vi "QinABCDQout.vi"(1 "ABCD":cluster{"A":dbl, "B":dbl, "C":dbl, "D":dbl} {"D" format="%.2f"; "C" format="%.2f"; "B" format="%.2f"; "A" format="%.2f"}, 2 "Q in":cdb format="%.2f") -> (0 "Q out":cdb format="%.2f")   [LabVIEW 2017]
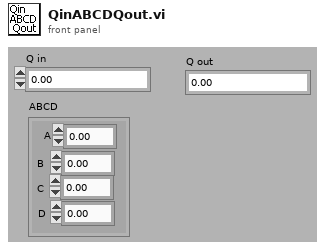
[diagram p1: front panel]
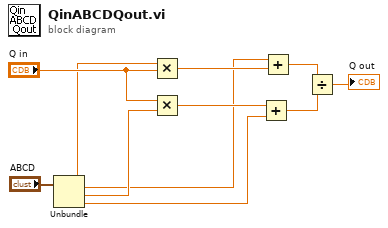
[diagram p0: block diagram]
diagram:
  n1 = Unbundle("ABCD") -> ("A"=w4:dbl, "B"=w2:dbl, "C"=w3:dbl, "D"=w1:dbl)
  n2 = Multiply(x=w4, y="Q in") -> (x*y=w10:cdb)
  n3 = Multiply(x="Q in", y=w3) -> (x*y=w9:cdb)
  n4 = Add(x=w9, y=w1) -> (x+y=w7:cdb)
  n5 = Add(x=w2, y=w10) -> (x+y=w8:cdb)
  n6 = Divide(x=w8, y=w7) -> (x/y=→"Q out":cdb)
